vi "Build Array.vi"() -> ()   [LabVIEW 2023]
panel:
  out "2DArray":u64[][](array[numeric])
  out "Out Array":u64[](array[numeric])
  out "Appended array":u64[](array[numeric])
  out "1D UArr":u64[](array[numeric])
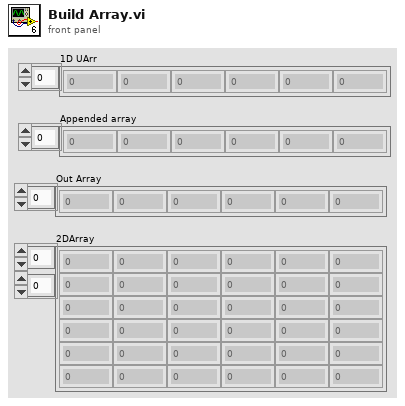
[diagram p1: front panel]
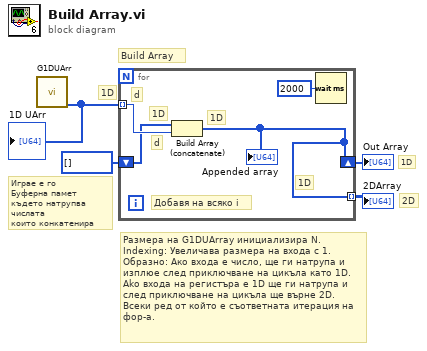
[diagram p0: block diagram]
diagram:
  # "1D"
  # "Играе е го\nБуферна памет\nкъдето натрупва числата\nкоито конкатенира"
  # "Build Array"
  # "2D"
  # "1D"
  # "Размера на G1DUArray инициализира N.\nIndexing: Увеличава размера на входа с 1.\nОбразно: Ако входа е число, ще ги натрупа и изплюе след приключване на цикъла като 1D. Ako входа на регистъра е 1D ще ги натрупа и след приключване на цикъла ще върне 2D. Всеки ред от който е съответната итерация на фор-а."
  n1 = call "G1DUArr.vi"() -> ("1D UArr"=w4:u64[])  [unwired: 11 in]
  "1D UArr" <- w4
  n2 = for {
    tunnel: w4 -> [w8] mode=indexing
    shift-right: [w5] -> w2
    shift-left: u64[] [] -> [w6]
    tunnel: [w5] -> w1 mode=indexing
    # "1D"
    # "1D"
    # "d"
    # "1D"
    # "d"
    # "Добавя на всяко i"
    n3 = Build Array (concatenate)(w6, w8) -> (w5:u64[])
    "Appended array" <- w5
    n4 = Wait (ms)(milliseconds to wait=u32 2000) -> ()  [unwired: 1 out]
  }
  "Out Array" <- w2
  "2DArray" <- w1
